vi "Follow Yaw.vi"() -> ()   [LabVIEW 2018]
panel:
  out "Follow Yaw":dbl
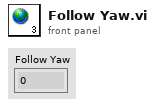
[diagram p1: front panel]
diagram:
